vi "HW Config_Check before Exit.vi"(11 "HW Configuration (each Station)":T1={"Results FilePath"=path "", "Analysis Parameters"={"Area"={"Lower Value"=10.0, "Upper Value"=500.0}, "Circle Filter Radius"={"Lower Value"=10.0, "Upper Value"=500.0}, "Edge Detection Threshold"=50}, "ROI Parameters"={"ROI size (in Radius)"={"Width"=1.0, "Height"=0.5}}}) -> (3 "T button?":bool)   [LabVIEW 2014]
uses:
  Custom Controls/TypeDef - System Configuration.ctl
  FileIO/TypeDef - File Actions.ctl
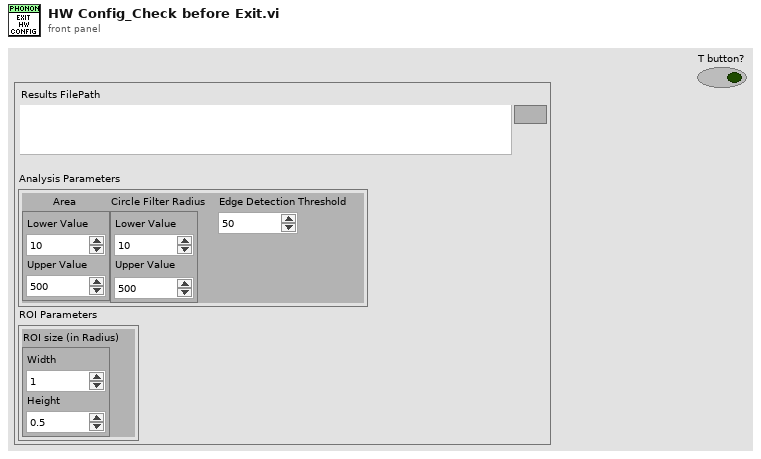
[diagram p1: front panel]
types:
  T1 = typedef "TypeDef - System Configuration.ctl" = cluster{"Results FilePath":path, "Analysis Parameters":cluster{"Area":cluster{"Lower Value":dbl, "Upper Value":dbl}, "Circle Filter Radius":cluster{"Lower Value":sgl, "Upper Value":sgl}, "Edge Detection Threshold":u16}, "ROI Parameters":cluster{"ROI size (in Radius)":cluster{"Width":dbl, "Height":dbl}}}
  T2 = typedef "TypeDef - File Actions.ctl" = enum16{"Read", "Write", "Get Current"}
  T3 = enum16{"Left Button", "Center Button", "Right Button", "Window Close"}
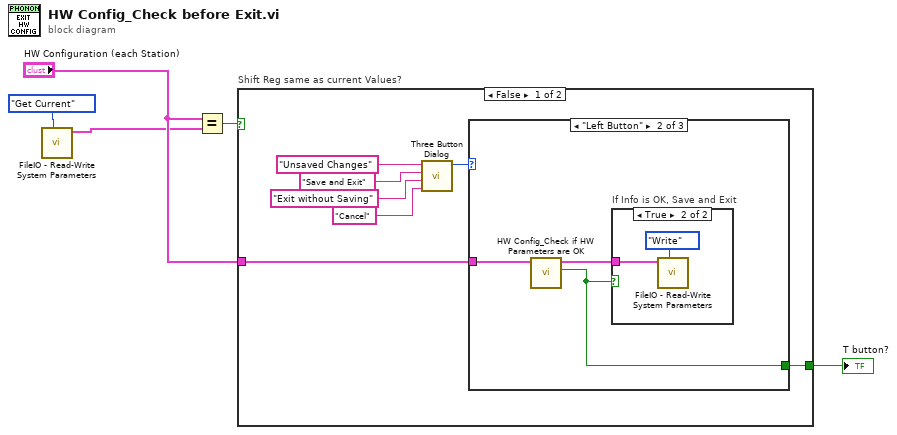
[diagram p0: block diagram]
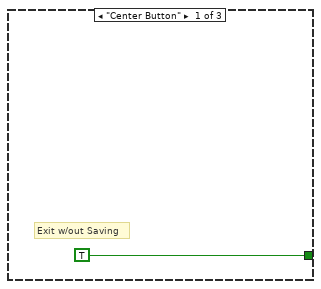
[diagram p2: hidden frame]
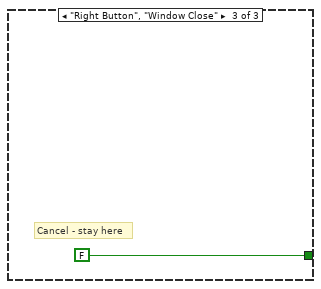
[diagram p4: hidden frame]
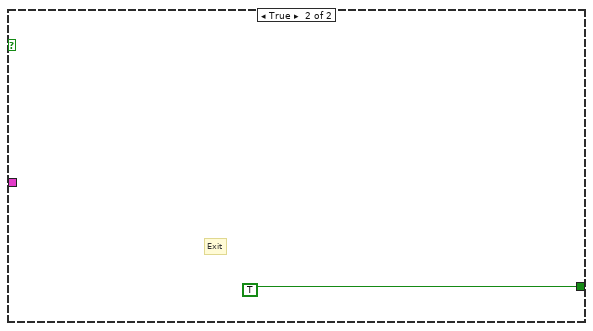
[diagram p5: hidden frame]
diagram:
  n1 = call "FileIO - Read-Write System Parameters.vi"("Action"=TypeDef_-_File_Actions."Get Current") -> ("System Parameters out"=w1:T1)  [unwired: 9 in, 1 out]
  n2 = Equal?(x="HW Configuration (each Station)", y=w1) -> (x = y?=w3:bool)
  n3 = case "Shift Reg same as current Values?" shown="False" w3 {
    tunnel: [w7 TRUE ("T button?")] -> w4
    tunnel: "HW Configuration (each Station)" -> [w6 _]
    frame False {
      n4 = call <vilib>:"Three Button Dialog.vi"("Right Button Text (\"Cancel\")"="Cancel" ("F button name (\"Cancel\")"), "Center Button Text (\"No\")"="Exit without Saving" ("F button name (\"Cancel\")"), "Left Button Text (\"Yes\")"="Save and Exit" ("T button name (\"OK\")"), "message"="Unsaved Changes") -> ("Which Button?"=w8:T3)  [unwired: 7 in]
      n5 = case shown="\"Left Button\"" w8 {
        tunnel: [TRUE ("T button?") w14 FALSE ("T button?")] -> w7
        tunnel: w6 -> [_ w15 _]
        frame "Center Button" {
          # "Exit w/out Saving"
        }
        frame "Left Button" {
          n6 = call "HW Config_Check if HW Parameters are OK.vi"("HW Configuration (each Station)"=w15) -> ("Info OK?"=w14:bool, "HW Configuration (each Station)"=w16:T1)  [unwired: 9 in]
          n7 = case "If Info is OK, Save and Exit" shown="True" w14 {
            tunnel: w16 -> [_ w18]
            frame False {
            }
            frame True {
              n8 = call "FileIO - Read-Write System Parameters.vi"("Action"=TypeDef_-_File_Actions."Write", "System Parameters in"=w18) -> ()  [unwired: 8 in, 2 out]
            }
          }
        }
        frame "Right Button", "Window Close" {
          # "Cancel - stay here"
        }
      }
    }
    frame True {
      # "Exit"
    }
  }
  "T button?" <- w4
